vi "时间转换.vi"(1 "数值":dbl) -> (0 "字符串":string)   [LabVIEW 2012]
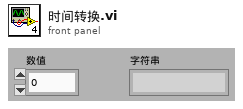
[diagram p1: front panel]
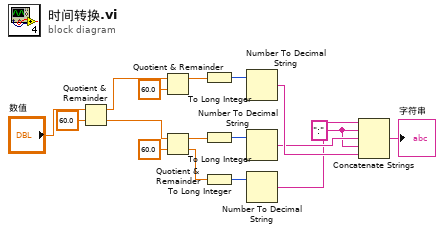
[diagram p0: block diagram]
diagram:
  w14 = ":" ("字符串")
  n1 = Quotient & Remainder(x="数值", y=60.0) -> (x-y*floor(x/y)=w4:dbl, floor(x/y)=w6:dbl)
  n2 = Quotient & Remainder(x=w4, y=60.0) -> (x-y*floor(x/y)=w12:dbl)  [unwired: 1 out]
  n3 = Quotient & Remainder(x=w6, y=60.0) -> (x-y*floor(x/y)=w10:dbl, floor(x/y)=w7:dbl)
  n4 = To Long Integer(number=w12) -> (32bit integer=w11:i32)
  n5 = To Long Integer(number=w10) -> (32bit integer=w9:i32)
  n6 = To Long Integer(number=w7) -> (32bit integer=w8:i32)
  n7 = Number To Decimal String(number=w11) -> (decimal integer string=w16:string)  [unwired: 1 in]
  n8 = Number To Decimal String(number=w9) -> (decimal integer string=w15:string)  [unwired: 1 in]
  n9 = Number To Decimal String(number=w8) -> (decimal integer string=w13:string)  [unwired: 1 in]
  n10 = Concatenate Strings(w13, w14, w15, w14, w16) -> (→"字符串":string)
